vi "BLM status.vi"(4 "error in (no error)":errorcluster, 6 "Motor Address":string="0", 7 "Port Address":refnum<visa-resource-name>) -> (0 "error out":errorcluster, 1 "Motor is moving":bool, 3 "Port Address Out":refnum<visa-resource-name>)   [LabVIEW 2019]
uses:
  BLM_IgnoreAlarms.vi
panel:
  out "BLM Status":bool[](array[boolean])
  out "Response":string
  # "SC command - Response Details:\nHex Value Status Code bit definition\n0001 Motor Enabled (Motor Disabled if this bit = 0)\n0002 Sampling (for Quick Tuner)\n0004 Drive Fault (check Alarm Code)\n0008 In Position (motor is in position)\n0010 Moving (motor is moving)\n0020 Jogging (currently in jog mode)\n0040 Stopping (in the process of stopping from a stop command)\n0080 Waiting (for an input)\n0100 Saving (parameter data is being saved)\n0200 Alarm present (check Alarm Code)\n0400 Homing (executing an SH command)\n0800 Wait Time (executing a WT command)\n1000 Wizard running (Timing Wizard is running)\n2000 Checking encoder (Timing Wizard is running)\n4000 Q Program is running\n8000 Initializing (happens at power up)"
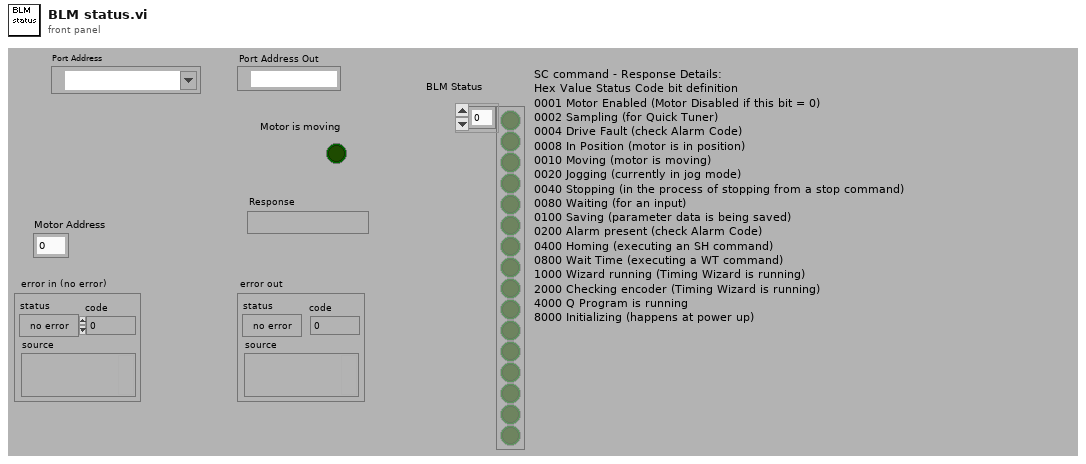
[diagram p1: front panel]
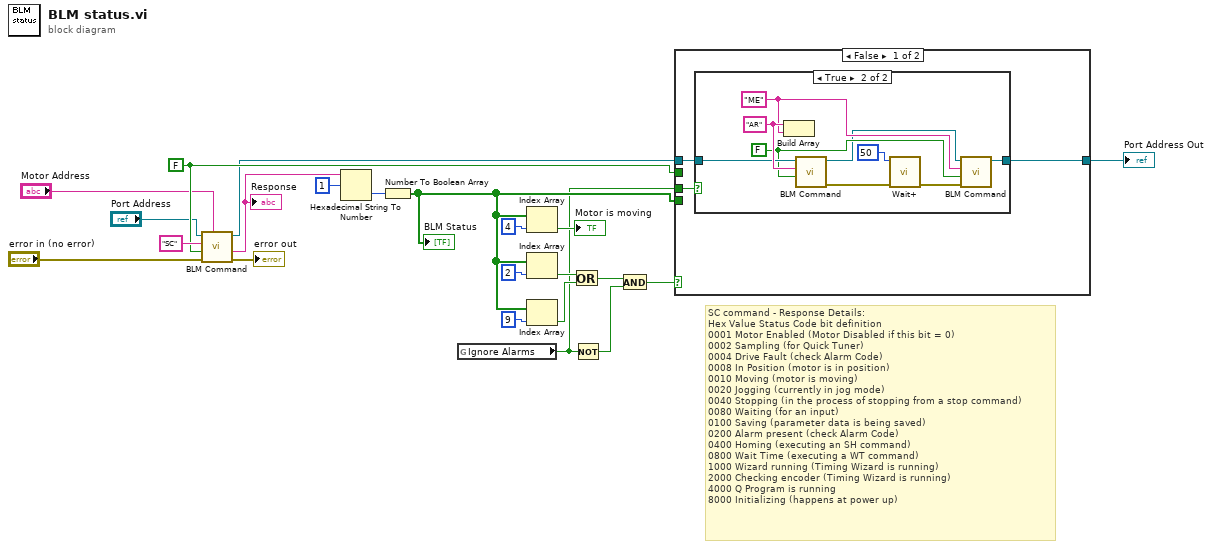
[diagram p0: block diagram]
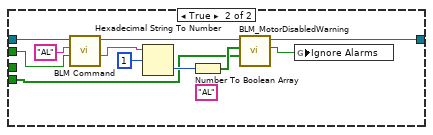
[diagram p3: hidden frame]
diagram:
  w9 = FALSE
  # "SC command - Response Details:\nHex Value Status Code bit definition\n0001 Motor Enabled (Motor Disabled if this bit = 0)\n0002 Sampling (for Quick Tuner)\n0004 Drive Fault (check Alarm Code)\n0008 In Position (motor is in position)\n0010 Moving (motor is moving)\n0020 Jogging (currently in jog mode)\n0040 Stopping (in the process of stopping from a stop command)\n0080 Waiting (for an input)\n0100 Saving (parameter data is being saved)\n0200 Alarm present (check Alarm Code)\n0400 Homing (executing an SH command)\n0800 Wait Time (executing a WT command)\n1000 Wizard running (Timing Wizard is running)\n2000 Checking encoder (Timing Wizard is running)\n4000 Q Program is running\n8000 Initializing (happens at power up)"
  n1 = call "BLM Command.vi"("Motor Address"="Motor Address", "error in (no error)"="error in (no error)", "Read Echo?"=w9, "Command"="SC", "Port Address"="Port Address") -> ("error out"=→"error out":errorcluster, "Response"=w19:string, "Port Address Out"=w1:refnum<visa-resource-name>)  [unwired: 1 in, 2 out]
  "Response" <- w19
  n2 = Hexadecimal String To Number(string=w19, offset=u32 1 ("initial scan location")) -> (number=w17:u32)  [unwired: 1 in, 1 out]
  n3 = Number To Boolean Array(number=w17) -> (Boolean array=w10:bool[])
  "BLM Status" <- w10
  n4 = global read "BLM_IgnoreAlarms.vi" "Ignore Alarms"() -> (w5:bool)
  n5 = Index Array(array=w10, index=4) -> (element=→"Motor is moving":bool)
  n6 = Index Array(array=w10, index=2) -> (element=w14:bool)
  n7 = Index Array(array=w10, index=9) -> (element=w13:bool)
  n8 = Or(x=w14, y=w13) -> (x .or. y?=w7:bool)
  n9 = Not(x=w5) -> (.not. x?=w6:bool)
  n10 = And(x=w7, y=w6) -> (x .and. y?=w8:bool)
  n11 = case shown="False" w8 {
    tunnel: w10 -> [_ w40]
    tunnel: w1 -> [w24 w39]
    tunnel: w9 -> [_ w46]
    tunnel: w5 -> [w25 _]
    tunnel: [w23 w36] -> w3
    frame False {
      n12 = case shown="True" w25 {
        tunnel: w24 -> [w26 w34]
        tunnel: [w26 w27] -> w23
        frame False {
        }
        frame True {
          w32 = "ME" ("Command")
          w33 = FALSE ("Read Echo?")
          w35 = "AR" ("Command")
          n13 = Build Array(w35, w32) -> ()  [unwired: 1 out]
          n14 = call "BLM Command.vi"("Read Echo?"=w33, "Command"=w35, "Port Address"=w34) -> ("error out"=w31:errorcluster, "Port Address Out"=w28:refnum<visa-resource-name>)  [unwired: 3 in, 3 out]
          n15 = call "Wait+.vi"("Error In"=w31, "milliseconds to wait"=u32 50) -> ("Error Out"=w30:errorcluster)  [unwired: 4 in, 1 out]
          n16 = call "BLM Command.vi"("error in (no error)"=w30, "Read Echo?"=w33, "Command"=w32, "Port Address"=w28) -> ("Port Address Out"=w27:refnum<visa-resource-name>)  [unwired: 2 in, 4 out]
        }
      }
    }
    frame True {
      (unwired) "AL" ("Command")
      n17 = call "BLM Command.vi"("Read Echo?"=w46, "Command"="AL", "Port Address"=w39) -> ("Response"=w42:string, "Port Address Out"=w37:refnum<visa-resource-name>)  [unwired: 3 in, 3 out]
      n18 = Hexadecimal String To Number(string=w42, offset=u32 1 ("initial scan location")) -> (number=w44:u32)  [unwired: 1 in, 1 out]
      n19 = Number To Boolean Array(number=w44) -> (Boolean array=w41:bool[])
      n20 = call "BLM_MotorDisabledWarning.vi"("BLM Status"=w40, "BLM Alarm Code"=w41, "Instrument Address"=w37) -> ("Ignore Alarms"=w38:bool, "Instrument Address Out"=w36:refnum<visa-resource-name>)  [unwired: 2 in, 1 out]
      n21 = global write "BLM_IgnoreAlarms.vi" "Ignore Alarms"(w38) -> ()
    }
  }
  "Port Address Out" <- w3
